vi "Move to XY or Z.vi"(8 "move type":enum16{"horizontal", "vertical"}(ring), 9 "Z":dbl[unit] min=0.0 max=12.0, 10 "position 1":T1, 11 "ID":i32) -> (2 "Response":string, 3 "ID out":i32)   [LabVIEW 2012]
uses:
  point.ctl
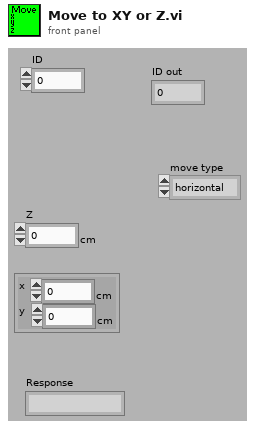
[diagram p1: front panel]
types:
  T1 = typedef "point.ctl" = cluster{"x":dbl[unit], "y":dbl[unit]}
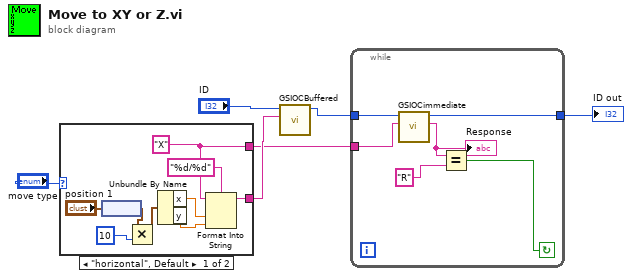
[diagram p0: block diagram]
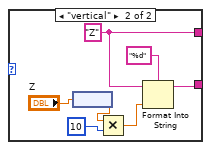
[diagram p2: hidden frame]
diagram:
  n1 = case shown="\"horizontal\", Default" "move type" {
    tunnel: [w15 w20] -> w5
    tunnel: [w14 w21] -> w3
    frame "horizontal", Default {
      w14 = "X" ("Command")
      n2 = node("position 1") -> (w9:cluster{"x":dbl, "y":dbl})
      n3 = Multiply(x=w9, y=10) -> (x*y=w7:cluster{"x":dbl, "y":dbl})
      n4 = Unbundle By Name(w7) -> ("x"=w11:dbl, "y"=w10:dbl)
      n5 = Format Into String(format string="%d/%d", initial string=w14, w11, w10) -> (resulting string=w15:string)  [unwired: 1 in, 1 out]
    }
    frame "vertical" {
      w21 = "Z" ("Command")
      n6 = node("Z") -> (w17:dbl)
      n7 = Multiply(x=w17, y=10) -> (x*y=w16:dbl)
      n8 = Format Into String(format string="%d", initial string=w21, w16) -> (resulting string=w20:string)  [unwired: 1 in, 1 out]
    }
  }
  n9 = call "GSIOCBuffered.vi"("Command"=w5, "ID"="ID") -> ("ID out"=w4:i32)  [unwired: 4 in, 1 out]
  n10 = while {
    tunnel: w4 -> [w28]
    tunnel: w3 -> [w27]
    tunnel: [w23] -> w2
    stop <- w24 continue-if-true
    n11 = call "GSIOCimmediate.vi"("Command"=w27, "ID"=w28) -> ("Response"=w25:string, "ID out"=w23:i32)  [unwired: 4 in]
    "Response" <- w25
    n12 = Equal?(x=w25, y="R" ("Response")) -> (x = y?=w24:bool)
  }
  "ID out" <- w2
